vi "Self-Test.vi"(8 "error in (no error)":errorcluster, 11 "VISA resource name":refnum<visa-resource-name>) -> (0 "error out":errorcluster, 2 "Test Pass?":bool, 3 "VISA resource name out":refnum<visa-resource-name>)   [LabVIEW 2011, in "Fluke 8508.lvlib"]
doc: "This VI runs the instrument's self test routine and returns the test results.\n\nNOTE: The self test can take several seconds to complete."
uses:
  Fluke 8508.lvlib
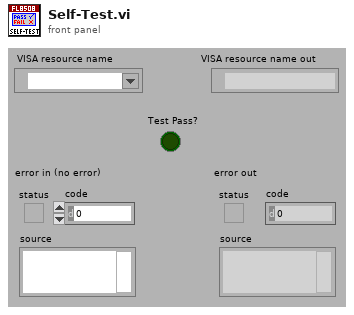
[diagram p1: front panel]
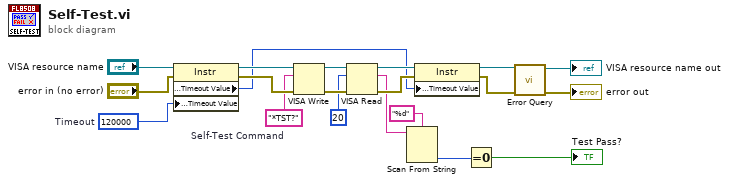
[diagram p0: block diagram]
diagram:
  w8 = u32 120000  # Timeout
  w4 = "*TST?"  # Self-Test Command
  n1 = property class="Instr"(reference="VISA resource name", error in="error in (no error)", "General Settings:Timeout Value"=w8) -> (reference out=w6:refnum<visa-resource-name>, error out=w7:errorcluster, "General Settings:Timeout Value"=w5:u32)
  n2 = VISA Write(VISA resource name=w6, write buffer=w4, error in (no error)=w7) -> (VISA resource name out=w18:refnum<visa-resource-name>, error out=w17:errorcluster)  [unwired: 1 out]
  n3 = VISA Read(VISA resource name=w18, byte count=u32 20 ("byte count (20)"), error in (no error)=w17) -> (VISA resource name out=w20:refnum<visa-resource-name>, read buffer=w13:string, error out=w19:errorcluster)  [unwired: 1 out]
  n4 = Scan From String(format string="%d", input string=w13) -> (output 1=w2:i32)  [unwired: 3 in, 3 out]
  n5 = property class="Instr"(reference=w20, error in=w19, "General Settings:Timeout Value"=w5) -> (reference out=w12:refnum<visa-resource-name>, error out=w11:errorcluster)
  n6 = Equal To 0?(x=w2) -> (x = 0?=→"Test Pass?":bool)
  n7 = call "Error Query.vi"("error in (no error)"=w11, "VISA resource name"=w12) -> ("error out"=→"error out":errorcluster, "VISA resource name out"=→"VISA resource name out":refnum<visa-resource-name>)  [unwired: 6 in, 2 out]
